vi "PH_Sixpack.contents.vi"   [LabVIEW 2014, in "PH_Sixpack.lvlib"]
doc: "This class is forseen to control a sixpack (Trinamic Motion Controller).\n\nThis class is part of the PHELIX device layer."
uses:
  PH_Sixpack.lvlib
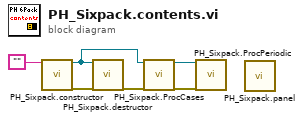
[diagram p0: block diagram]
diagram:
  n1 = call "PH_Sixpack.constructor.vi"("name"="") -> ("i ref out"=w1:refnum<vi>, "error out"=w3:errorcluster)  [unwired: 16 in, 1 out]
  n2 = call "PH_Sixpack.destructor.vi"("i ref in"=w1, "error in"=w3) -> ("error out"=w4:errorcluster)  [unwired: 17 in]
  n3 = call "PH_Sixpack.ProcCases.vi"("i ref in"=w1, "error in"=w4) -> ("i ref out"=w6:refnum<vi>, "error out"=w5:errorcluster)  [unwired: 15 in, 1 out]
  n4 = call "PH_Sixpack.ProcPeriodic.vi"("i ref in"=w6, "error in"=w5) -> ()  [unwired: 15 in, 3 out]
  n5 = call "PH_Sixpack.panel.vi"() -> ()  [unwired: 19 in, 1 out]
